vi "Initialize.vi"(8 "error in (no error)":errorcluster, 11 "PLC in":refnum<class "MB PLC Client.lvclass">) -> (0 "error out":errorcluster, 3 "PLC out":refnum<class "MB PLC Client.lvclass">)   [LabVIEW 2018, in "MB PLC Client.lvlib" / "MB PLC Client.lvclass"]
uses:
  MB PLC Client.lvclass
  MB PLC Client.lvclass/MB PLC Client.ctl
  <vilib>/Plasmionique/MB Master/MB_Master_Serial/MB_Master_Serial.lvclass
  C:/Program Files (x86)/National Instruments/LabVIEW 2018/vi.lib/Plasmionique/MB Master/MB_Master/MB_Master.lvclass
  <vilib>/Plasmionique/MB Master/MB_Master_TCP/MB_Master_TCP.lvclass
  <vilib>/Plasmionique/MB Master/MB_Master/MB_Master.lvclass
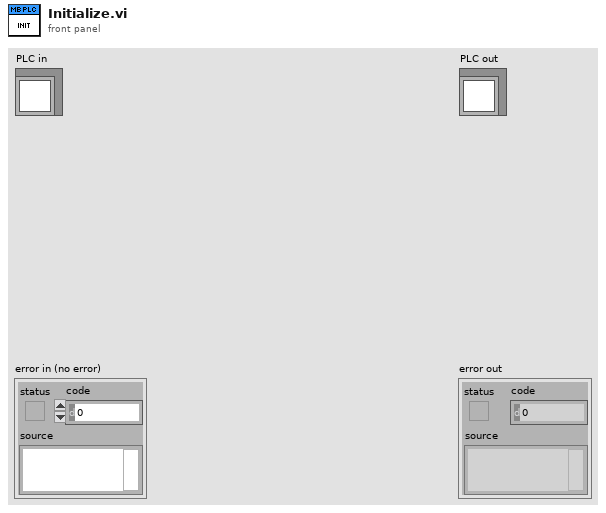
[diagram p1: front panel]
types:
  T1 = cluster{"baud rate (bps)":u32, "stop bits":u16, "parity":u16, "flow control":u16, "timeout":u32, "retries":i32}
  T2 = typedef "MB PLC Client.lvlib/Serial Config_Cluster.ctl" = cluster{"COM Port":string, "Slave ID":u8, "baud rate (bps)":u32, "Mode":enum16{"RTU", "ASCII"}, "Parity":u16, "Flow Control":u16, "Timeout":u32, "Retries":u8, "Stop Bits":u16}
  T3 = typedef "MB PLC Client.lvlib/TCP Config_Cluster.ctl" = cluster{"IP Address":string, "Port":u16, "Slave ID":i8, "Timeout":i32}
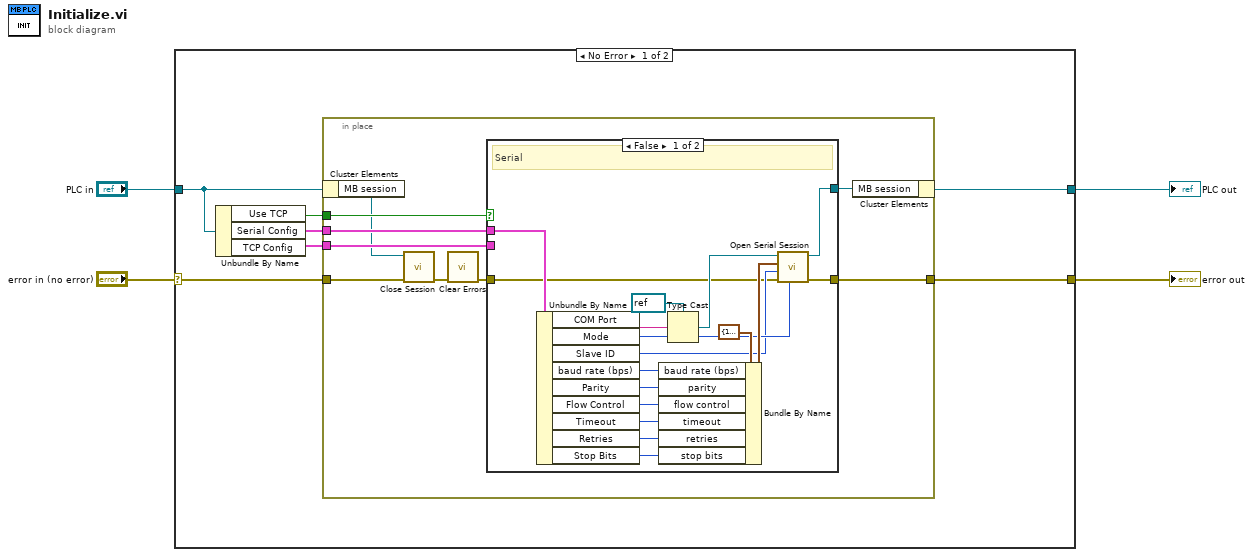
[diagram p0: block diagram]
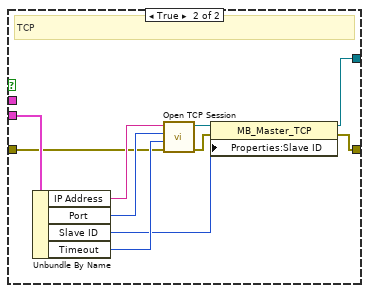
[diagram p2: hidden frame]
diagram:
  n1 = case shown="No Error" "error in (no error)" {
    selector: "error in (no error)" -> [w5 w48]
    tunnel: [w11 w48] -> w4
    tunnel: "PLC in" -> [w10 w49]
    tunnel: [w9 w49] -> w2
    frame No Error {
      n2 = Unbundle By Name(w10) -> ("Use TCP"=w8:bool, "Serial Config"=w7:T2, "TCP Config"=w6:T3)
      n3 = in-place {
        in-place-border: w5 -> [w16]
        in-place-border: [w20] -> w11
        in-place-border: w8 -> [w19]
        in-place-border: w7 -> [w18]
        in-place-border: w6 -> [w17]
        n4 = in-place-cluster #1(w10) -> ("MB session"=w13:refnum<class "MB_Master.lvclass">)
        n5 = call-dynamic "Close Session.vi"("error in (no error)"=w16, "MB session in"=w13) -> ("error out"=w15:errorcluster)  [unwired: 9 in]
        n6 = call <vilib>:"Clear Errors.vi"("error in (no error)"=w15) -> ("error out"=w14:errorcluster)  [unwired: 5 in, 1 out]
        n7 = case shown="False" w19 {
          tunnel: w14 -> [w21 w38]
          tunnel: [w28 w40] -> w20
          tunnel: [w24 w42] -> w12
          tunnel: w18 -> [w23 _]
          tunnel: w17 -> [_ w47]
          frame False {
            # "Serial"
            n8 = Unbundle By Name(w23) -> ("COM Port"=w22:string, "Mode"=w29:enum16{"RTU", "ASCII"}, "Slave ID"=w27:u8, "baud rate (bps)"=w31:u32, "Parity"=w32:u16, "Flow Control"=w33:u16, "Timeout"=w34:u32, "Retries"=w25:u8, "Stop Bits"=w26:u16)
            n9 = Bundle By Name(cluster=T1 {"baud rate (bps)"=19200, "stop bits"=10, "parity"=0, "flow control"=0, "timeout"=1000, "retries"=1} ("Serial Config"), "baud rate (bps)"=w31, "parity"=w32, "flow control"=w33, "timeout"=w34, "retries"=w25, "stop bits"=w26) -> (w30:T1)
            n10 = Type Cast(type=refnum<visa-resource-name> refnum ("VISA resource"), x=w22) -> (*(type *) &x=w36:refnum<visa-resource-name>)
            n11 = call <vilib>:"Open Serial Session.vi"("Mode (RTU)"=w29, "Error in"=w21, "Slave ID"=w27, "Serial Config"=w30, "VISA Resource"=w36) -> ("Error out"=w28:errorcluster, "MB_Serial session"=w24:refnum<class "MB_Master_Serial.lvclass">)  [unwired: 5 in]
          }
          frame True {
            # "TCP"
            n12 = Unbundle By Name(w47) -> ("IP Address"=w46:string, "Port"=w45:u16, "Slave ID"=w39:i8, "Timeout"=w44:i32)
            n13 = call <vilib>:"Open TCP Session.vi"("error in (no error)"=w38, "Timeout (10000)"=w44, "Port (502)"=w45, "IP Address"=w46) -> ("error out"=w41:errorcluster, "MB_TCP session"=w43:refnum<class "MB_Master_TCP.lvclass">)  [unwired: 6 in]
            n14 = property class="MB_Master_TCP"(reference=w43, error in=w41, "Properties:Slave ID"=w39) -> (reference out=w42:refnum<class "MB_Master_TCP.lvclass">, error out=w40:errorcluster)
          }
        }
        n15 = in-place-cluster #1("MB session"=w12) -> (w9:refnum<class "MB PLC Client.lvclass">)
      }
    }
    frame Error {
    }
  }
  "error out" <- w4
  "PLC out" <- w2
